vi "PLC_ReadData(Boolean).vi"(8 "error in (no error)":errorcluster, 10 "LogicName":string, 11 "Message Enqueuer":refnum<class "Message Enqueuer.lvclass">) -> (0 "error out":errorcluster, 3 "data":bool)   [LabVIEW 2025, in "PLC_API.lvlib"]
uses:
  PLC_API.lvlib
  <vilib>/ActorFramework/Message Enqueuer/Message Enqueuer.lvclass
  PLC_Module/PLC_Module Messages/ReadData Msg/ReadData Msg.lvclass/ReadData Msg.ctl
  <vilib>/ActorFramework/Message Enqueuer/Message Enqueuer.lvclass/Message Enqueuer.ctl
  <vilib>/ActorFramework/Message Enqueuer/Enqueue.vi
  PLC_Module/PLC_Module Messages/ReadData Msg/ReadData Msg.lvclass
  C:/Program Files (x86)/National Instruments/LabVIEW 2025/vi.lib/ActorFramework/Message/Message.lvclass
  <vilib>/ActorFramework/Message Priority Queue/Priority Enqueue.vi
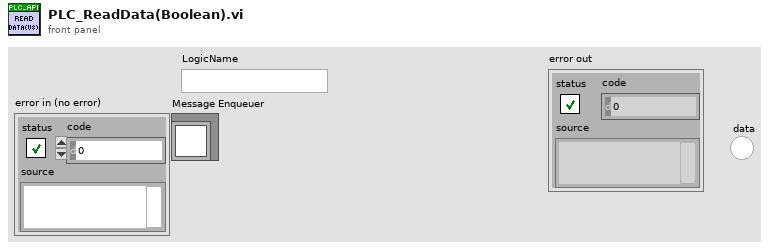
[diagram p1: front panel]
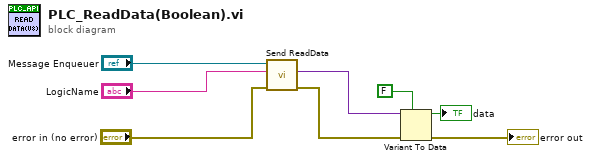
[diagram p0: block diagram]
diagram:
  n1 = call "Send ReadData.vi"("error in (no error)"="error in (no error)", "LogicName"="LogicName", "Message Enqueuer"="Message Enqueuer") -> ("error out"=w4:errorcluster, "Data"=w5:variant)  [unwired: 6 in, 1 out]
  n2 = Variant To Data(error in=w4, type=FALSE, Variant=w5) -> (data=→"data":bool, error out=→"error out":errorcluster)
